vi "Begin.vi"(8 "error in":errorcluster) -> (0 "error out":errorcluster)   [LabVIEW 2017]
doc: "Called before other user functions, this VI is expected to open initial I/O refnums, load in file data, and do all program initialization. Notice that the <B>error out</B> terminal is simply used for data flow. Wiring it to other structures or subVIs ensures that this VI runs first."
uses:
  <vilib>/Rock Robotics/WPI/DriverStation/WPI_DriverStationRobotMode2.ctl
  Robot Global Data.vi
  <vilib>/Rock Robotics/Network Tables/NT Write String Array.vi
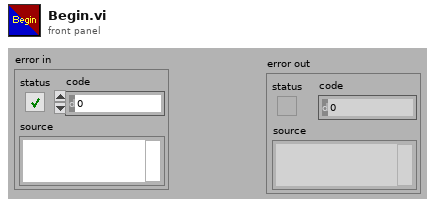
[diagram p1: front panel]
types:
  T1 = typedef "WPI_DriverStationRobotMode2.ctl" = enum16{"Autonomous Disabled", "Autonomous Enabled", "Teleop Disabled", "Teleop Enabled", "Disconnected", "Finish", "Test Disabled", "Test Enabled", "Emergency Stopped"}
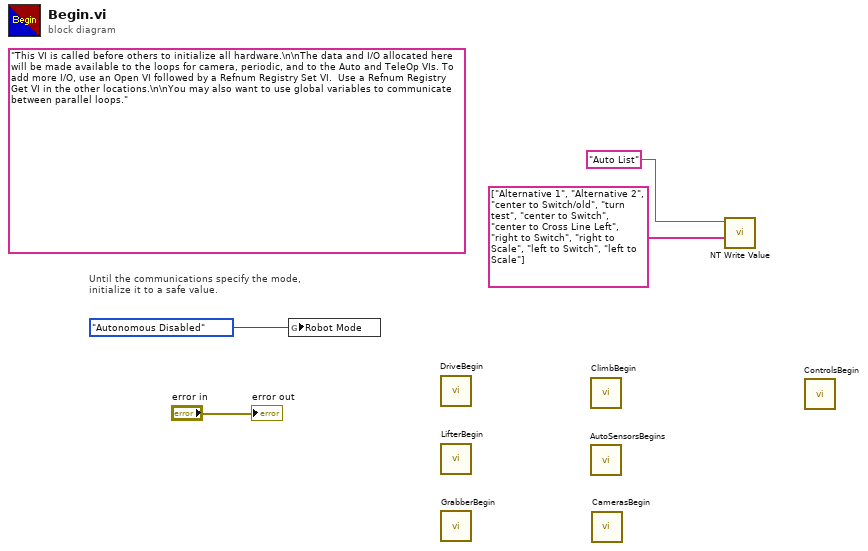
[diagram p0: block diagram]
diagram:
  (unwired) "This VI is called before others to initialize all hardware.\n\nThe data and I/O allocated here will be made available to the loops for camera, periodic, and to the Auto and TeleOp VIs. To add more I/O, use an Open VI followed by a Refnum Registry Set VI.  Use a Refnum Registry Get VI in the other locations.\n\nYou may also want to use global variables to communicate between parallel loops."
  # "Until the communications specify the mode,\ninitialize it to a safe value."
  n1 = global write "Robot Global Data.vi" "Robot Mode"(WPI_DriverStationRobotMode2."Autonomous Disabled" ("Robot Mode")) -> ()
  n2 = call "DriveBegin.vi"() -> ()  [unwired: 12 in]
  n3 = call "LifterBegin.vi"() -> ()  [unwired: 12 in]
  n4 = call "GrabberBegin.vi"() -> ()  [unwired: 12 in]
  n5 = call "ClimbBegin.vi"() -> ()  [unwired: 12 in]
  n6 = call "AutoSensorsBegins.vi"() -> ()  [unwired: 12 in]
  n7 = call "CamerasBegin.vi"() -> ()  [unwired: 12 in]
  n8 = call-poly <vilib>:"NT Write Value.vi"("String Array"=string[] ["Alternative 1", "Alternative 2", "center to Switch/old", "turn test", "center to Switch", "center to Cross Line Left", "right to Switch", "right to Scale", "left to Switch", "left to Scale"], "Name"="Auto List") -> ()  [unwired: 9 in, 1 out]
  n9 = call "ControlsBegin.vi"() -> ()  [unwired: 12 in]
  "error out" <- "error in"
